vi "test-PID-input-output.vi"(8 "error in (no error)":errorcluster) -> (0 "error out":errorcluster, 3 "All Passed":bool)   [LabVIEW 2019]
uses:
  <vilib>/Rock Robotics/WPI/ThirdParty/JAS_Junk/TrajLib/TypeDef/PID_CONTROLLER.ctl
  <vilib>/Rock Robotics/WPI/ThirdParty/JAS_Junk/TrajLib/PIDController_NewPeriod.vi
  <vilib>/Rock Robotics/WPI/ThirdParty/JAS_Junk/TrajLib/PIDController_SetSetpoint.vi
  <vilib>/Rock Robotics/WPI/ThirdParty/JAS_Junk/TrajLib/PIDController_Calculate_PV.vi
  <vilib>/Rock Robotics/SystemInterfaces/NetworkCommunication/NetComm_UsageReport_report.vi
  <vilib>/Rock Robotics/WPI/ThirdParty/JAS_Junk/TrajLib/ControllerUtil_GetModulusError.vi
  <vilib>/Rock Robotics/WPI/ThirdParty/JAS_Junk/TrajLib/Globals/Util_LibraryGlobals.vi
  <vilib>/Rock Robotics/WPI/ThirdParty/JAS_Junk/TrajLib/Trajectory_Library.lvlib
panel:
  out "T5 Passed":bool
  out "T4 Passed":bool
  out "T3 Passed":bool
  out "T2 Passed":bool
  out "T1 Passed":bool
  out "T0 Passed":bool
  out "T0 PID CTRL":T1={"Kp"=0.0, "Ki"=0.0, "Kd"=0.0, "Period"=0.0, "Max_Integral"=0.0, "Min_Integral"=0.0, "Max_Input"=0.0, "Min_Input"=0.0, "Continuous"=FALSE, "PositionError"=0.0, "VelocityError"=0.0, "PrevError"=0.0, "Total_Integral"=0.0, "PositionTolerance"=0.0, "VelocityTolerance"=0.0, "SetPoint"=0.0, "Kf"=0.0, "Prev_Deriv"=0.0, "Prev_Deriv 2"=0.0, "DerivativeFilter"=FALSE, "Min_Output"=-9.99e+35, "Max_Output"=9.9e+35, "Prev_F_P"=0.0, "Prev_F_P_2"=0.0, "AntiWindupActive"=FALSE, "Measurement"=0.0, "IntegralZone"=9.9e+30} {"IntegralZone" format="%16_6e"; "Measurement" format="%16_6e"; "Prev_F_P_2" format="%16_6e"; "Prev_F_P" format="%16_6e"; "Max_Output" format="%16_6e"; "Min_Output" format="%16_6e"; "Prev_Deriv 2" format="%16_6e"; "Prev_Deriv" format="%16_6e"; "Kf" format="%16_6e"; "SetPoint" format="%16_6e"; "VelocityTolerance" format="%16_6e"; "PositionTolerance" format="%16_6e"; "Total_Integral" format="%16_6e"; "PrevError" format="%16_6e"; "VelocityError" format="%16_6e"; "PositionError" format="%16_6e"; "Min_Input" format="%16_6e"; "Max_Input" format="%16_6e"; "Min_Integral" format="%16_6e"; "Max_Integral" format="%16_6e"; "Period" format="%16_6e"; "Kd" format="%16_6e"; "Ki" format="%16_6e"; "Kp" format="%16_6e"}
  out "T3 -- Output =":dbl
  out "T2 -- Output  = -0.01":dbl
  out "T1 -- Output  = -0.1":dbl
  out "T0 -- Output < 0":dbl
  # "PID Input Output"
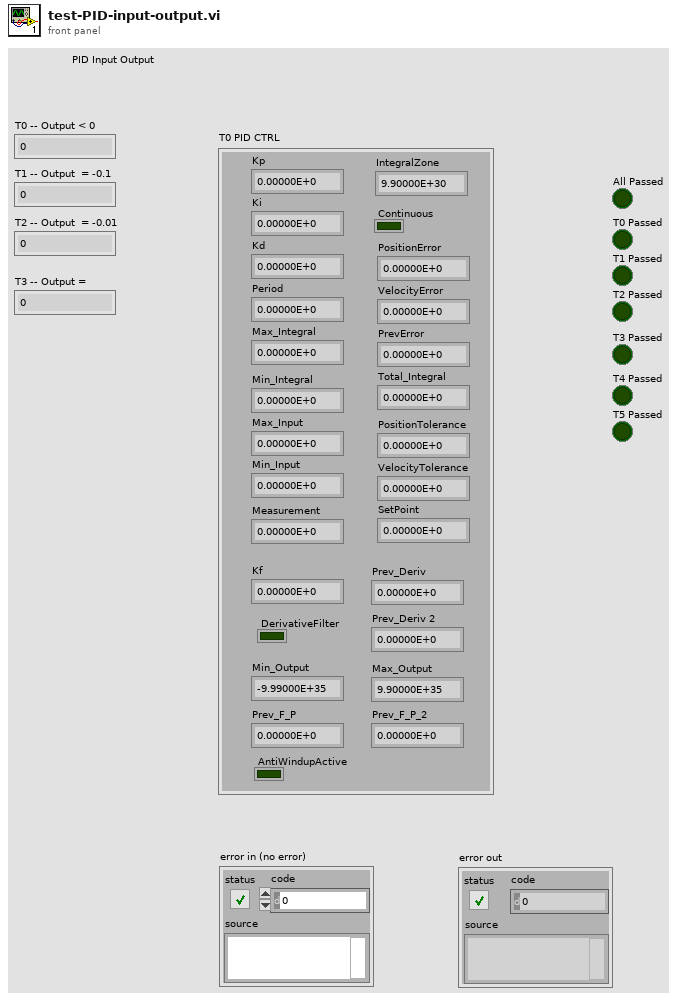
[diagram p1: front panel]
types:
  T1 = typedef "Trajectory_Library.lvlib/PID_CONTROLLER.ctl" = cluster{"Kp":dbl, "Ki":dbl, "Kd":dbl, "Period":dbl, "Max_Integral":dbl, "Min_Integral":dbl, "Max_Input":dbl, "Min_Input":dbl, "Continuous":bool, "PositionError":dbl, "VelocityError":dbl, "PrevError":dbl, "Total_Integral":dbl, "PositionTolerance":dbl, "VelocityTolerance":dbl, "SetPoint":dbl, "Kf":dbl, "Prev_Deriv":dbl, "Prev_Deriv 2":dbl, "DerivativeFilter":bool, "Min_Output":dbl, "Max_Output":dbl, "Prev_F_P":dbl, "Prev_F_P_2":dbl, "AntiWindupActive":bool, "Measurement":dbl, "IntegralZone":dbl}
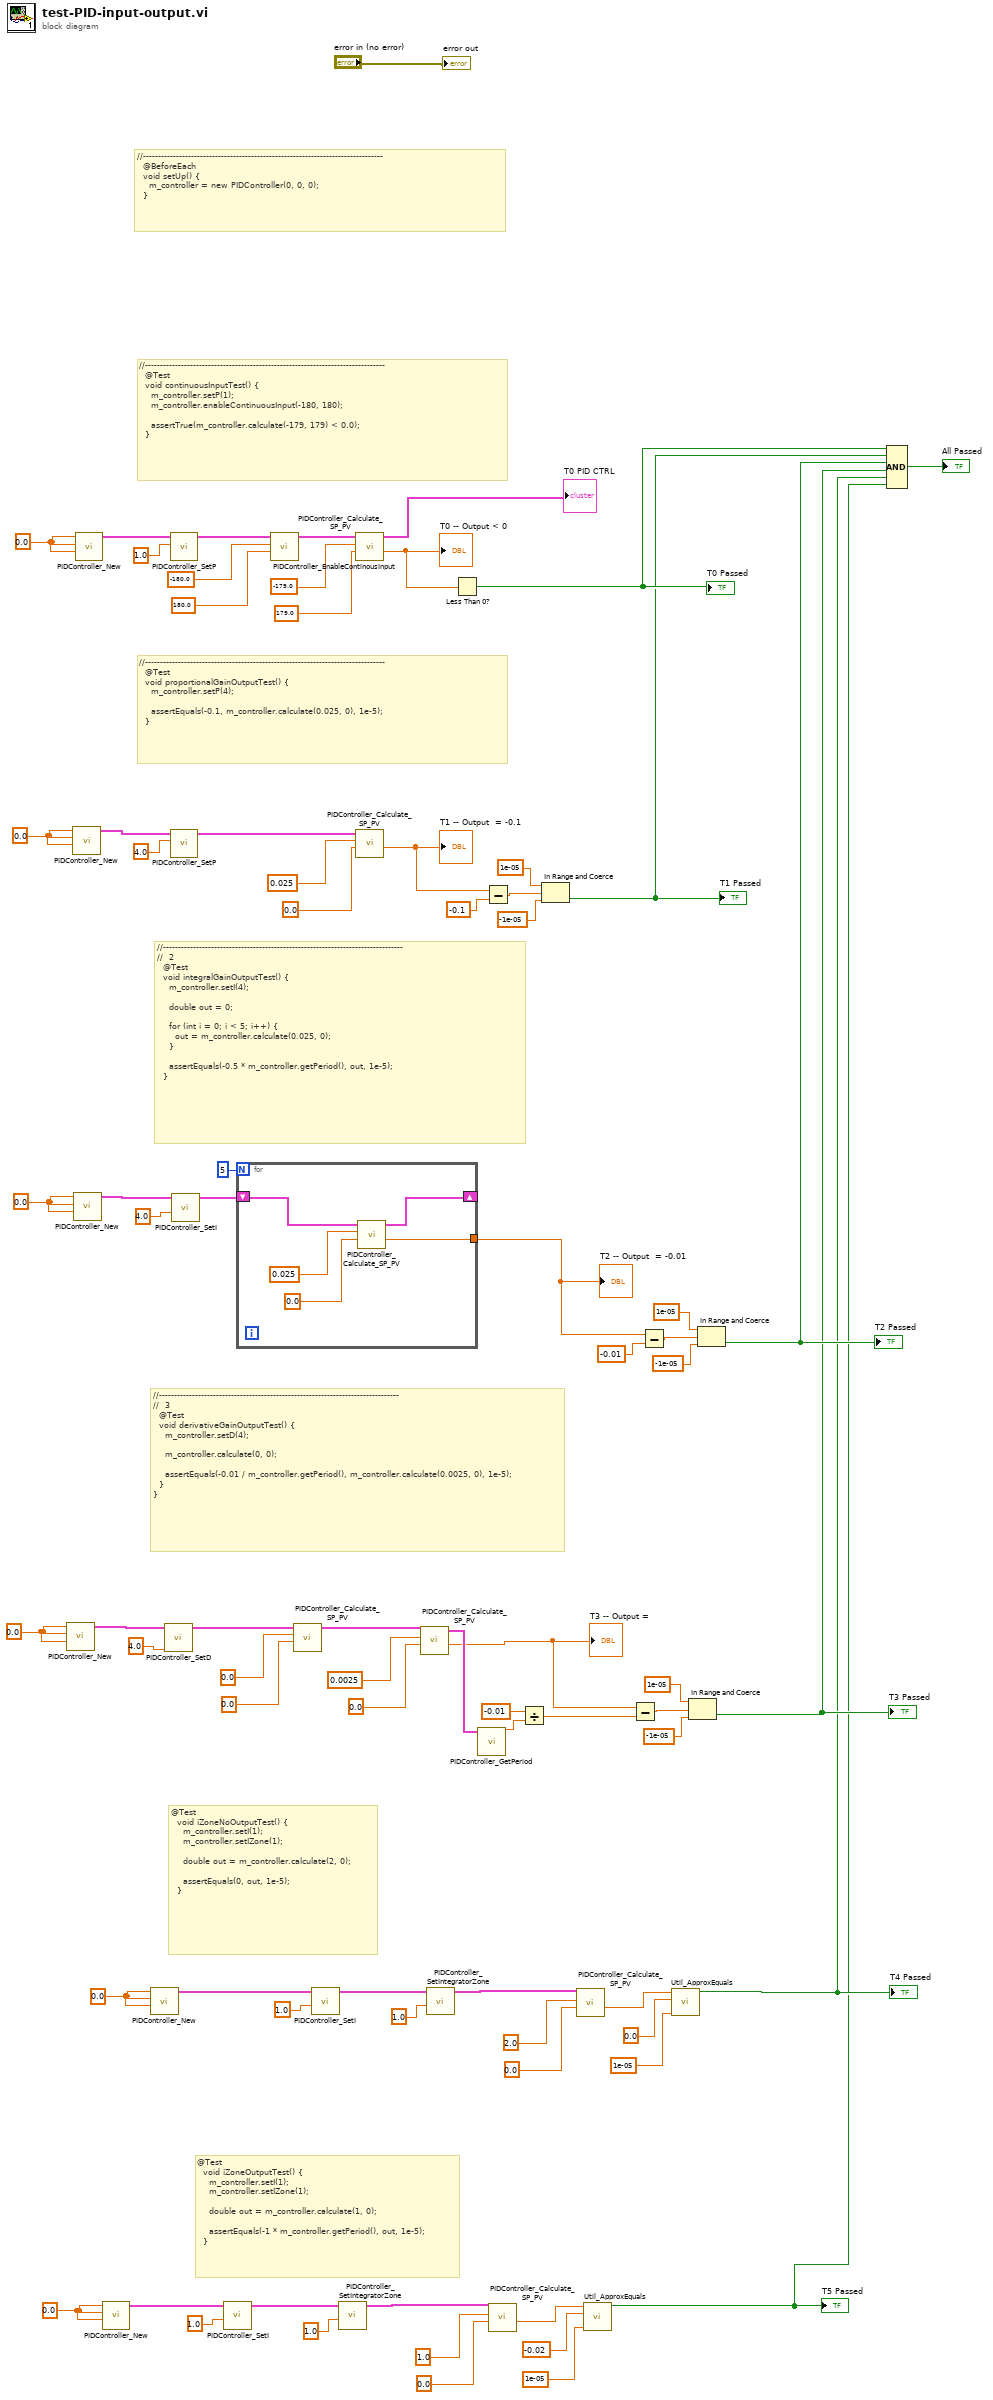
[diagram p0: block diagram]
diagram:
  w5 = 0.0 ("Kp")
  w7 = 0.0 ("Kp")
  w9 = 0.0 ("Kp")
  w11 = 0.0 ("Kp")
  w13 = 0.0 ("Kp")
  w79 = 0.0 ("Kp")
  # "@Test\n  void iZoneOutputTest() {\n    m_controller.setI(1);\n    m_controller.setIZone(1);\n\n    double out = m_controller.calculate(1, 0);\n\n    assertEquals(-1 * m_controller.getPeriod(), out, 1e-5);\n  }"
  # "@Test\n  void iZoneNoOutputTest() {\n    m_controller.setI(1);\n    m_controller.setIZone(1);\n\n    double out = m_controller.calculate(2, 0);\n\n    assertEquals(0, out, 1e-5);\n  }"
  # "//--------------------------------------------------------------------------------\n//  3\n  @Test\n  void derivativeGainOutputTest() {\n    m_controller.setD(4);\n\n    m_controller.calculate(0, 0);\n\n    assertEquals(-0.01 / m_controller.getPeriod(), m_controller.calculate(0.0025, 0), 1e-5);\n  }\n}"
  # "//--------------------------------------------------------------------------------\n//  2\n  @Test\n  void integralGainOutputTest() {\n    m_controller.setI(4);\n\n    double out = 0;\n\n    for (int i = 0; i < 5; i++) {\n      out = m_controller.calculate(0.025, 0);\n    }\n\n    assertEquals(-0.5 * m_controller.getPeriod(), out, 1e-5);\n  }"
  # "//--------------------------------------------------------------------------------\n  @Test\n  void proportionalGainOutputTest() {\n    m_controller.setP(4);\n\n    assertEquals(-0.1, m_controller.calculate(0.025, 0), 1e-5);\n  }"
  # "//--------------------------------------------------------------------------------\n  @BeforeEach\n  void setUp() {\n    m_controller = new PIDController(0, 0, 0);\n  }"
  # "//--------------------------------------------------------------------------------\n  @Test\n  void continuousInputTest() {\n    m_controller.setP(1);\n    m_controller.enableContinuousInput(-180, 180);\n\n    assertTrue(m_controller.calculate(-179, 179) < 0.0);\n  }"
  n1 = call <vilib>:"PIDController_New.vi"("Kd"=w9, "Ki"=w9, "Kp"=w9) -> ("PID_CONTROLLER"=w8:T1)  [unwired: 8 in]
  n2 = call <vilib>:"PIDController_New.vi"("Kd"=w5, "Ki"=w5, "Kp"=w5) -> ("PID_CONTROLLER"=w4:T1)  [unwired: 8 in]
  n3 = call <vilib>:"PIDController_New.vi"("Kd"=w7, "Ki"=w7, "Kp"=w7) -> ("PID_CONTROLLER"=w6:T1)  [unwired: 8 in]
  n4 = call <vilib>:"PIDController_New.vi"("Kd"=w79, "Ki"=w79, "Kp"=w79) -> ("PID_CONTROLLER"=w3:T1)  [unwired: 8 in]
  n5 = call <vilib>:"PIDController_New.vi"("Kd"=w11, "Ki"=w11, "Kp"=w11) -> ("PID_CONTROLLER"=w10:T1)  [unwired: 8 in]
  n6 = call <vilib>:"PIDController_New.vi"("Kd"=w13, "Ki"=w13, "Kp"=w13) -> ("PID_CONTROLLER"=w12:T1)  [unwired: 8 in]
  n7 = call <vilib>:"PIDController_SetD.vi"("Kd"=4.0 ("Kp"), "in PID_CONTROLLER"=w8) -> ("out PID_CONTROLLER"=w63:T1)  [unwired: 9 in]
  n8 = call <vilib>:"PIDController_SetP.vi"("Kp"=1.0, "in PID_CONTROLLER"=w3) -> ("out PID_CONTROLLER"=w77:T1)  [unwired: 9 in]
  n9 = call <vilib>:"PIDController_SetP.vi"("Kp"=4.0, "in PID_CONTROLLER"=w4) -> ("out PID_CONTROLLER"=w68:T1)  [unwired: 9 in]
  n10 = call <vilib>:"PIDController_SetI.vi"("Ki"=4.0 ("Kp"), "in PID_CONTROLLER"=w6) -> ("out PID_CONTROLLER"=w66:T1)  [unwired: 9 in]
  n11 = call <vilib>:"PIDController_SetI.vi"("Ki"=1.0 ("Kp"), "in PID_CONTROLLER"=w10) -> ("out PID_CONTROLLER"=w21:T1)  [unwired: 9 in]
  n12 = for {
    N: 5 -> [_]
    tunnel: [w82] -> w46
    shift-right: [w80] -> _
    shift-left: w66 -> [w81]
    n13 = call <vilib>:"PIDController_Calculate_SP_PV.vi"("SP-SetPoint"=0.0, "PV-Measurement"=0.025, "in PID_CONTROLLER"=w81) -> ("CO-ControlOutput"=w82:dbl, "out PID_CONTROLLER"=w80:T1)  [unwired: 7 in]
  }
  "T2 -- Output  = -0.01" <- w46
  n14 = call <vilib>:"PIDController_EnableContinousInput.vi"("MaxInput"=180.0, "MinInput"=-180.0, "in PID_CONTROLLER"=w77) -> ("out PID_CONTROLLER"=w74:T1)  [unwired: 8 in]
  n15 = call <vilib>:"PIDController_Calculate_SP_PV.vi"("SP-SetPoint"=0.0, "PV-Measurement"=0.0, "in PID_CONTROLLER"=w63) -> ("out PID_CONTROLLER"=w58:T1)  [unwired: 7 in, 1 out]
  n16 = call <vilib>:"PIDController_SetI.vi"("Ki"=1.0 ("Kp"), "in PID_CONTROLLER"=w12) -> ("out PID_CONTROLLER"=w30:T1)  [unwired: 9 in]
  n17 = call <vilib>:"PIDController_SetIntegratorZone.vi"("IntegratorZone"=1.0, "in PID_CONTROLLER"=w21) -> ("out PID_CONTROLLER"=w17:T1)  [unwired: 9 in]
  n18 = call <vilib>:"PIDController_Calculate_SP_PV.vi"("SP-SetPoint"=179.0, "PV-Measurement"=-179.0, "in PID_CONTROLLER"=w74) -> ("CO-ControlOutput"=w56:dbl, "out PID_CONTROLLER"=→"T0 PID CTRL":T1)  [unwired: 7 in]
  "T0 -- Output < 0" <- w56
  n19 = call <vilib>:"PIDController_Calculate_SP_PV.vi"("SP-SetPoint"=0.0, "PV-Measurement"=0.025, "in PID_CONTROLLER"=w68) -> ("CO-ControlOutput"=w54:dbl)  [unwired: 7 in, 1 out]
  "T1 -- Output  = -0.1" <- w54
  n20 = call <vilib>:"PIDController_Calculate_SP_PV.vi"("SP-SetPoint"=0.0, "PV-Measurement"=0.0025, "in PID_CONTROLLER"=w58) -> ("CO-ControlOutput"=w38:dbl, "out PID_CONTROLLER"=w45:T1)  [unwired: 7 in]
  "T3 -- Output =" <- w38
  n21 = call <vilib>:"PIDController_SetIntegratorZone.vi"("IntegratorZone"=1.0, "in PID_CONTROLLER"=w30) -> ("out PID_CONTROLLER"=w26:T1)  [unwired: 9 in]
  n22 = Less Than 0?(x=w56) -> (x < 0?=w37:bool)
  "T0 Passed" <- w37
  n23 = call <vilib>:"PIDController_GetPeriod.vi"("in PID_CONTROLLER"=w45) -> ("Period"=w44:dbl)  [unwired: 10 in]
  n24 = Subtract(x=w54, y=-0.1) -> (x-y=w51:dbl)
  n25 = call <vilib>:"PIDController_Calculate_SP_PV.vi"("SP-SetPoint"=0.0, "PV-Measurement"=1.0, "in PID_CONTROLLER"=w17) -> ("CO-ControlOutput"=w16:dbl)  [unwired: 7 in, 1 out]
  n26 = Divide(x=-0.01, y=w44) -> (x/y=w39:dbl)
  n27 = In Range and Coerce(upper limit=1e-05, x=w51, lower limit=-1e-05 ("upper limit")) -> (In Range?=w36:bool)  [unwired: 1 out]
  "T1 Passed" <- w36
  n28 = call <vilib>:"PIDController_Calculate_SP_PV.vi"("SP-SetPoint"=0.0, "PV-Measurement"=2.0, "in PID_CONTROLLER"=w26) -> ("CO-ControlOutput"=w25:dbl)  [unwired: 7 in, 1 out]
  n29 = call <vilib>:"Util_ApproxEquals.vi"("Tolerance"=1e-05, "Value 2"=-0.02, "Value 1"=w16) -> ("ApproxEquals"=w1:bool)  [unwired: 8 in]
  "T5 Passed" <- w1
  n30 = Subtract(x=w38, y=w39) -> (x-y=w41:dbl)
  n31 = Subtract(x=w46, y=-0.01) -> (x-y=w48:dbl)
  n32 = call <vilib>:"Util_ApproxEquals.vi"("Tolerance"=1e-05, "Value 2"=0.0, "Value 1"=w25) -> ("ApproxEquals"=w2:bool)  [unwired: 8 in]
  "T4 Passed" <- w2
  n33 = In Range and Coerce(upper limit=1e-05, x=w41, lower limit=-1e-05 ("upper limit")) -> (In Range?=w33:bool)  [unwired: 1 out]
  "T3 Passed" <- w33
  n34 = In Range and Coerce(upper limit=1e-05, x=w48, lower limit=-1e-05 ("upper limit")) -> (In Range?=w34:bool)  [unwired: 1 out]
  "T2 Passed" <- w34
  n35 = Compound Arithmetic op=AND(w37, w36, w34, w33, w2, w1) -> (→"All Passed":bool)
  "error out" <- "error in (no error)"
